vi "1-3.vi"() -> ()   [LabVIEW 2018]
panel:
  out "最小值":dbl
  out "最大值":dbl
  out "随机数":dbl
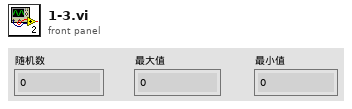
[diagram p1: front panel]
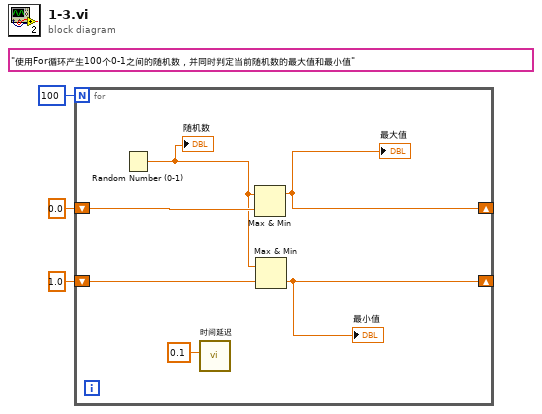
[diagram p0: block diagram]
diagram:
  (unwired) "使用For循环产生100个0-1之间的随机数，并同时判定当前随机数的最大值和最小值"
  n1 = for {
    N: 100 -> [_]
    shift-right: [w8] -> _
    shift-left: 0.0 -> [w9]
    shift-right: [w5] -> _
    shift-left: 1.0 -> [w6]
    n2 = Random Number (0-1)() -> (number: 0 to 1=w7:dbl)
    "随机数" <- w7
    n3 = call "时间延迟"("Delay Time (s)"=0.1) -> ()  [unwired: 10 in, 1 out]
    n4 = Max & Min(x=w7, y=w9) -> (max(x,y)=w8:dbl)  [unwired: 1 out]
    "最大值" <- w8
    n5 = Max & Min(x=w7, y=w6) -> (min(x,y)=w5:dbl)  [unwired: 1 out]
    "最小值" <- w5
  }
